vi "Update Channel Data.vi"(0 "Sequencer in":refnum<class "Sequencer.lvclass">, 1 "Channel Enququer":refnum<class "Message Enqueuer.lvclass">, 2 "ChannelData":refnum<class "ChannelData.lvclass">, 3 "error in (no error)":errorcluster) -> (7 "Sequencer out":refnum<class "Sequencer.lvclass">, 10 "error out":errorcluster)   [LabVIEW 2015, in "Sequencer.lvlib" / "Sequencer.lvclass"]
uses:
  Sequencer.lvclass
  <vilib>/ActorFramework/Message Enqueuer/Message Enqueuer.lvclass
  Channel/ChannelData.lvclass
  Sequencer.lvclass/Sequencer.ctl
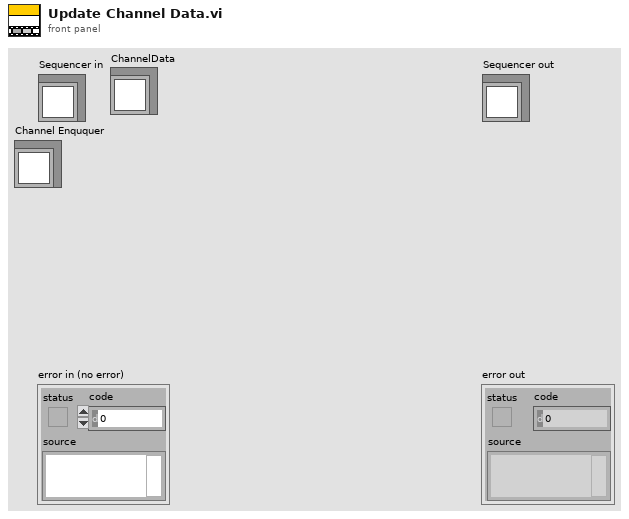
[diagram p1: front panel]
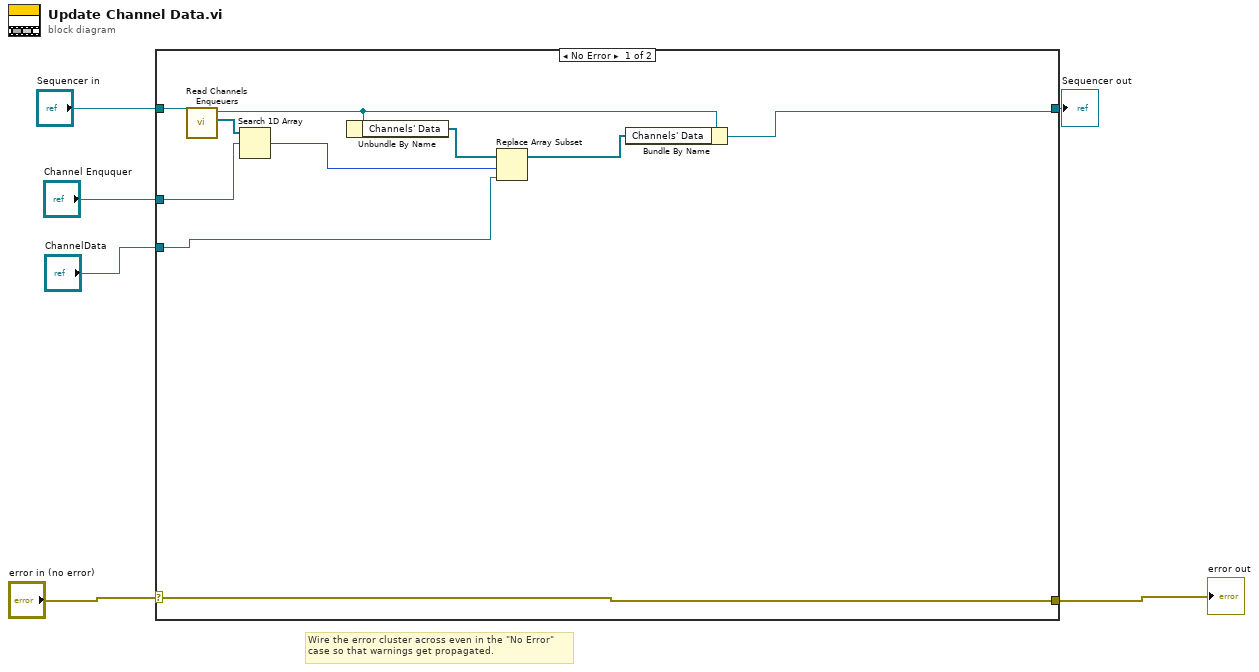
[diagram p0: block diagram]
diagram:
  # "Wire the error cluster across even in the \"No Error\"\ncase so that warnings get propagated."
  n1 = case shown="No Error" "error in (no error)" {
    selector: "error in (no error)" -> [w16 w18]
    tunnel: [w16 w18] -> w5
    tunnel: [w8 w17] -> w3
    tunnel: "Sequencer in" -> [w15 w17]
    tunnel: "Channel Enququer" -> [w13 _]
    tunnel: "ChannelData" -> [w10 _]
    frame No Error {
      n2 = call "Read Channels Enqueuers.vi"("Sequencer in"=w15) -> ("Channels Enqueuers"=w14:refnum<class "Message Enqueuer.lvclass">[], "Sequencer out"=w9:refnum<class "Sequencer.lvclass">)  [unwired: 8 in, 1 out]
      n3 = Search 1D Array(1D array=w14, element=w13) -> (index of element=w11:i32)  [unwired: 1 in]
      n4 = Unbundle By Name(w9) -> ("Channels' Data"=w12:refnum<class "ChannelData.lvclass">[])
      n5 = Replace Array Subset(array=w12, new element=w10, index=w11) -> (w7:refnum<class "ChannelData.lvclass">[])
      n6 = Bundle By Name(cluster=w9, "Channels' Data"=w7) -> (w8:refnum<class "Sequencer.lvclass">)
    }
    frame Error {
    }
  }
  "error out" <- w5
  "Sequencer out" <- w3
